vi "NovaTech409A_Set_Initial_TableMode.vi"(2 "error in (no error)":errorcluster, 3 "Novatech Ramp":T1 {"3 phase" format="%#.5f"; "2 phase" format="%#.5f"; "3 Power [dBm]" format="%#.5f"; "3 Freq. [MHz]" format="%#_5e"; "2 Power [dBm]" format="%#.5f"; "2 Freq. [MHz]" format="%#_5e"}, 4 "VISA resource name":refnum<visa-resource-name>="COM1") -> (0 "error out":errorcluster, 1 "VISA resource name out":refnum<visa-resource-name>="COM1")   [LabVIEW 2012, in "Novatech 409A.lvlib"]
doc: "This VI sets the \"static\" setting of all 4 novatech channels. Channels 0 and 1 are assumed to be ramping and the static values are set to the first value in the dynamic array. This way if modes switch the novatech is still set to a sane setting on all channels."
uses:
  Novatech 409A.lvlib
  EvapRampNumericTriggered.ctt
  Controls.llb/Controls.lvlib
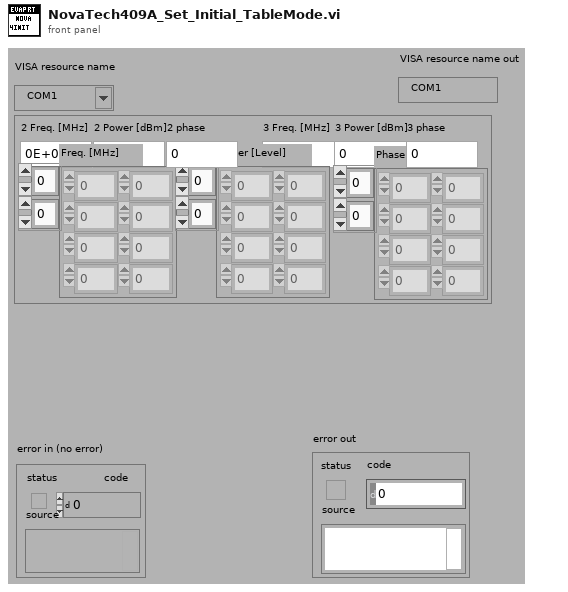
[diagram p1: front panel]
types:
  T1 = typedef "Controls.lvlib/EvapRampNumericTriggered.ctt" = cluster{"Freq. [MHz]":dbl[][], "Power [Level]":u16[][], "Phase":u16[][], "2 Freq. [MHz]":dbl, "2 Power [dBm]":u16, "2 phase":u16, "3 Freq. [MHz]":dbl, "3 Power [dBm]":u16, "3 phase":u16}
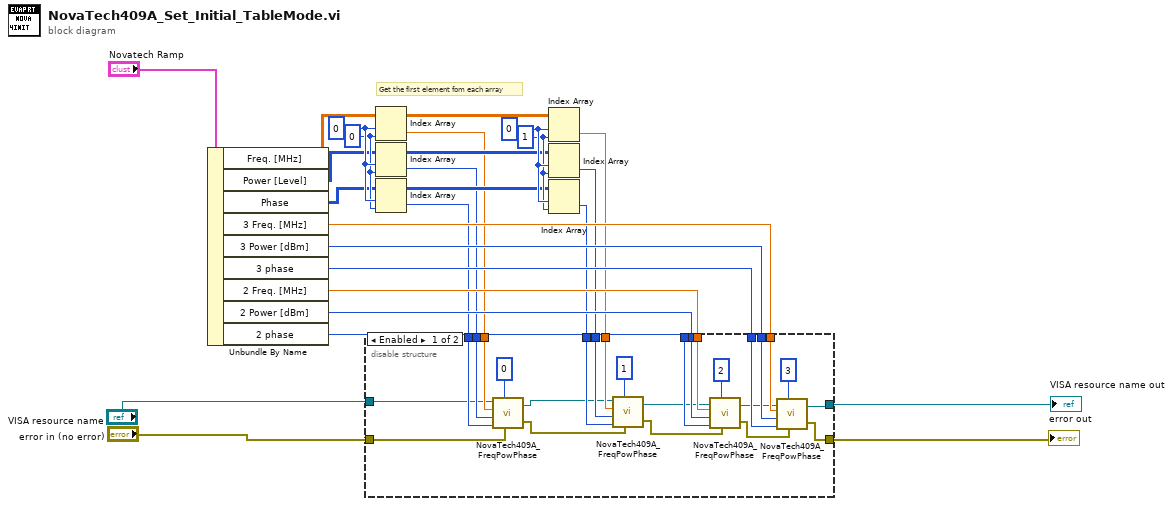
[diagram p0: block diagram]
diagram:
  w11 = 1 ("disabled index (col)")
  w12 = 0 ("index (row)")
  w13 = 0 ("disabled index (col)")
  w14 = 0 ("index (row)")
  # "Get the first element fom each array"
  n1 = Unbundle By Name("Novatech Ramp") -> ("Freq. [MHz]"=w10:dbl[][], "Power [Level]"=w9:u16[][], "Phase"=w8:u16[][], "3 Freq. [MHz]"=w21:dbl, "3 Power [dBm]"=w22:u16, "3 phase"=w19:u16, "2 Freq. [MHz]"=w23:dbl, "2 Power [dBm]"=w24:u16, "2 phase"=w20:u16)
  n2 = Index Array(array=w10, index (row)=w14, index (col)=w13) -> (element=w7:dbl)
  n3 = Index Array(array=w9, index (row)=w14, index (col)=w13) -> (element=w6:u16)
  n4 = Index Array(array=w8, index (row)=w14, index (col)=w13) -> (element=w5:u16)
  n5 = Index Array(array=w10, index (row)=w12, index (col)=w11) -> (element=w2:dbl)
  n6 = Index Array(array=w9, index (row)=w12, index (col)=w11) -> (element=w3:u16)
  n7 = Index Array(array=w8, index (row)=w12, index (col)=w11) -> (element=w4:u16)
  n8 = disable-structure shown="Enabled" {
    disable-tunnel: w24 -> [w50 _]
    disable-tunnel: w23 -> [w49 _]
    disable-tunnel: w22 -> [w48 _]
    disable-tunnel: w21 -> [w47 _]
    disable-tunnel: w20 -> [w44 _]
    disable-tunnel: w19 -> [w43 _]
    disable-tunnel: "error in (no error)" -> [w29 w51]
    disable-tunnel: "VISA resource name" -> [w34 w52]
    disable-tunnel: [w25 w51] -> w15
    disable-tunnel: w7 -> [w40 _]
    disable-tunnel: w6 -> [w39 _]
    disable-tunnel: w5 -> [w38 _]
    disable-tunnel: w4 -> [w37 _]
    disable-tunnel: w3 -> [w36 _]
    disable-tunnel: w2 -> [w35 _]
    disable-tunnel: [w30 w52] -> w1
    frame Enabled {
      n9 = call "NovaTech409A_FreqPowPhase.vi"("error in (no error)"=w29, "Channel (0-3)"=u8 0, "Phase"=w38, "Power"=w39, "Freq"=w40, "VISA resource name"=w34) -> ("error out"=w28:errorcluster, "VISA resource name out"=w33:refnum<visa-resource-name>)
      n10 = call "NovaTech409A_FreqPowPhase.vi"("error in (no error)"=w28, "Channel (0-3)"=u8 1, "Phase"=w37, "Power"=w36, "Freq"=w35, "VISA resource name"=w33) -> ("error out"=w27:errorcluster, "VISA resource name out"=w32:refnum<visa-resource-name>)
      n11 = call "NovaTech409A_FreqPowPhase.vi"("error in (no error)"=w27, "Channel (0-3)"=u8 2, "Phase"=w44, "Power"=w50, "Freq"=w49, "VISA resource name"=w32) -> ("error out"=w26:errorcluster, "VISA resource name out"=w31:refnum<visa-resource-name>)
      n12 = call "NovaTech409A_FreqPowPhase.vi"("error in (no error)"=w26, "Channel (0-3)"=u8 3, "Phase"=w43, "Power"=w48, "Freq"=w47, "VISA resource name"=w31) -> ("error out"=w25:errorcluster, "VISA resource name out"=w30:refnum<visa-resource-name>)
    }
    frame Disabled {
    }
  }
  "error out" <- w15
  "VISA resource name out" <- w1
